vi "global variables.vi"() -> ()   [LabVIEW 2023]
panel:
  in  "Pressure":dbl
  in  "O2":dbl
  in  "Ar":dbl
  in  "DC":dbl
  in  "REF":dbl
  in  "FWD":dbl
  in  "CT":dbl
  in  "CL":dbl
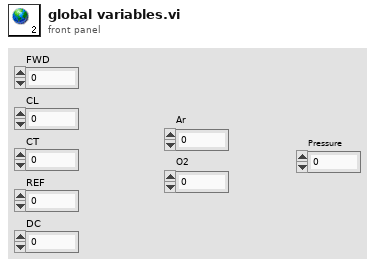
[diagram p1: front panel]
diagram:
